vi "read_csv_StoreTrajectory_FGV.vi"(8 "Sample Time\nSeconds":dbl, 9 "inTRAJECTORY":T6 {"States"."POSE"."ROTATION"."SIN" format="%13.4f"; "States"."POSE"."ROTATION"."COS" format="%13.4f"; "States"."POSE"."ROTATION"."VALUE" format="%13.4f"; "States"."POSE"."TRANSLATION"."Y" format="%14.3f"; "States"."POSE"."TRANSLATION"."X" format="%14.3f"; "TotalTImeSecs" format="%20.3f"}, 11 "Command":T5(ring)) -> (1 "outTRAJECTORY":T6 {"States"."POSE"."ROTATION"."SIN" format="%13.4f"; "States"."POSE"."ROTATION"."COS" format="%13.4f"; "States"."POSE"."ROTATION"."VALUE" format="%13.4f"; "States"."POSE"."TRANSLATION"."Y" format="%14.3f"; "States"."POSE"."TRANSLATION"."X" format="%14.3f"; "TotalTImeSecs" format="%20.3f"}, 3 "outTrajectoryState":T1={"TimeSeconds"=0.0, "Velocity"=0.0, "Acceleration"=0.0, "POSE"={"TRANSLATION"={"X"=0.0, "Y"=0.0}, "ROTATION"={"VALUE"=0.0, "COS"=1.0, "SIN"=0.0}}, "Curvature"=0.0} {"POSE"."ROTATION"."SIN" format="%13.4f"; "POSE"."ROTATION"."COS" format="%13.4f"; "POSE"."ROTATION"."VALUE" format="%13.4f"; "POSE"."TRANSLATION"."Y" format="%14.3f"; "POSE"."TRANSLATION"."X" format="%14.3f"})   [LabVIEW 2019]
uses:
  <vilib>/Rock Robotics/WPI/ThirdParty/JAS_Junk/TrajLib/TypeDef/TRAJECTORY.ctl
  <vilib>/Rock Robotics/WPI/ThirdParty/JAS_Junk/TrajLib/TypeDef/TRAJ_STATE.ctl
  <vilib>/Rock Robotics/WPI/ThirdParty/JAS_Junk/TrajLib/TypeDef/POSE2D.ctl
  <vilib>/Rock Robotics/WPI/ThirdParty/JAS_Junk/TrajLib/TypeDef/TRANSLATION2D.ctl
  <vilib>/Rock Robotics/WPI/ThirdParty/JAS_Junk/TrajLib/TypeDef/ROTATION2D.ctl
  <vilib>/Rock Robotics/WPI/ThirdParty/JAS_Junk/TrajLib/Trajectory_Library.lvlib
panel:
  # "This is purposefully \n\nNOT re-entrant."
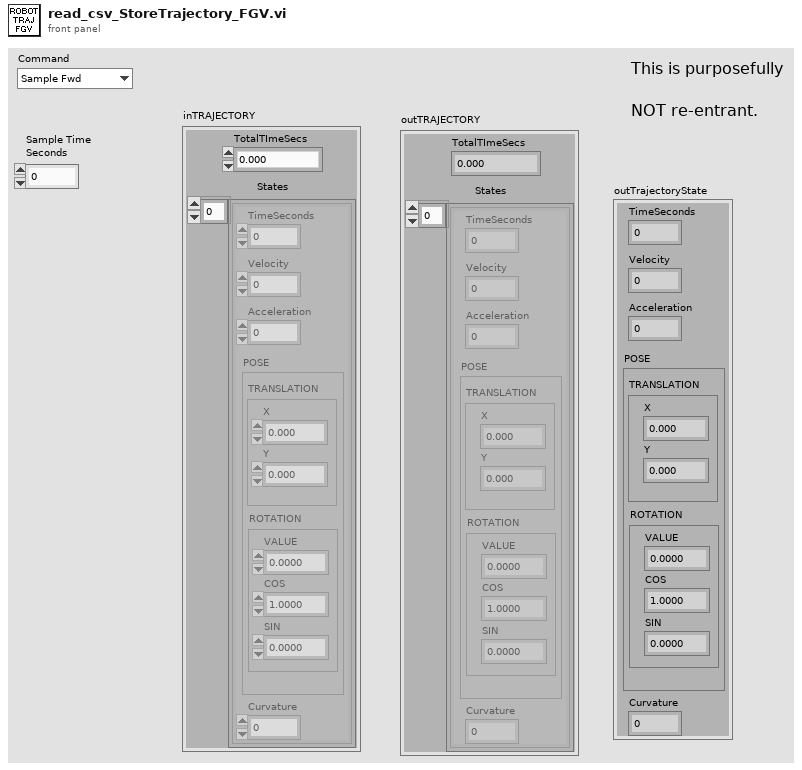
[diagram p1: front panel]
types:
  T1 = typedef "Trajectory_Library.lvlib/TRAJ_STATE.ctl" = cluster{"TimeSeconds":dbl, "Velocity":dbl, "Acceleration":dbl, "POSE":T2, "Curvature":dbl}
  T2 = typedef "Trajectory_Library.lvlib/POSE2D.ctl" = cluster{"TRANSLATION":T3, "ROTATION":T4}
  T3 = typedef "Trajectory_Library.lvlib/TRANSLATION2D.ctl" = cluster{"X":dbl, "Y":dbl}
  T4 = typedef "Trajectory_Library.lvlib/ROTATION2D.ctl" = cluster{"VALUE":dbl, "COS":dbl, "SIN":dbl}
  T5 = enum16{"Sample Fwd", "Sample Rev", "Read Traj", "Write Traj"}
  T6 = typedef "Trajectory_Library.lvlib/TRAJECTORY.ctl" = cluster{"TotalTImeSecs":dbl, "States":T1[]}
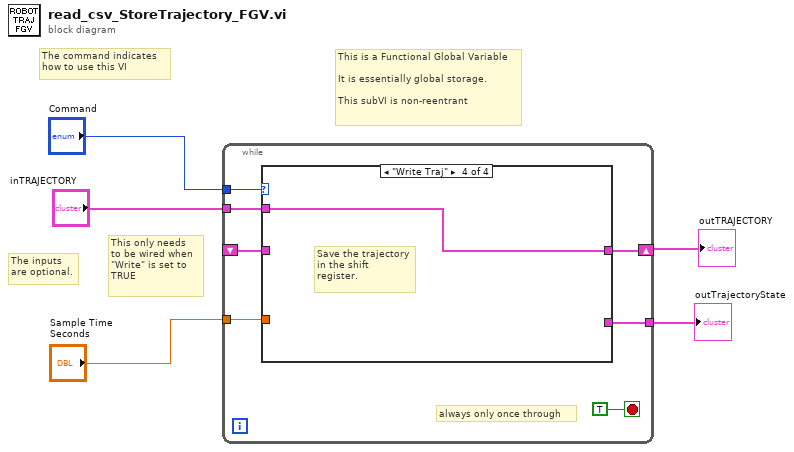
[diagram p0: block diagram]
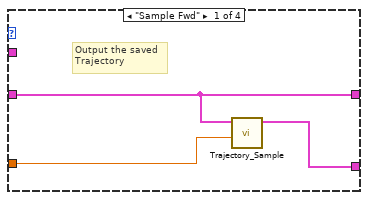
[diagram p2: hidden frame]
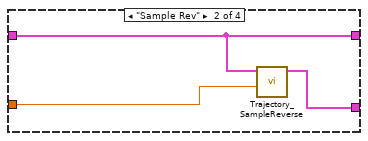
[diagram p3: hidden frame]
diagram:
  # "This only needs\nto be wired when\n\"Write\" is set to\nTRUE"
  # "The command indicates\nhow to use this VI"
  # "The inputs \nare optional."
  # "This is a Functional Global Variable\n\nIt is essentially global storage.\n\nThis subVI is non-reentrant"
  n1 = while {
    tunnel: "Command" -> [w11]
    tunnel: "inTRAJECTORY" -> [w9]
    shift-right: [w10] -> w5
    shift-left: _ -> [w8]
    tunnel: "Sample Time\nSeconds" -> [w7]
    tunnel: [w6] -> w1
    stop <- TRUE stop-if-true
    # "always only once through"
    n2 = case shown="\"Write Traj\"" w11 {
      tunnel: [w15 w18 w19 w20] -> w10
      tunnel: w9 -> [_ _ _ w20]
      tunnel: w8 -> [w15 w18 w19 _]
      tunnel: w7 -> [w14 w17 _ _]
      tunnel: [w13 w16 _ _] -> w6
      frame "Sample Fwd" {
        # "Output the saved\nTrajectory"
        n3 = call <vilib>:"Trajectory_Sample.vi"("Time"=w14, "InputTRAJECTORY"=w15) -> ("OutputTRAJ_STATE"=w13:T1)  [unwired: 9 in]
      }
      frame "Sample Rev" {
        n4 = call <vilib>:"Trajectory_SampleReverse.vi"("Time"=w17, "InputTRAJECTORY"=w18) -> ("OutputTRAJ_STATE"=w16:T1)  [unwired: 9 in]
      }
      frame "Read Traj" {
      }
      frame "Write Traj" {
        # "Save the trajectory\nin the shift \nregister."
      }
    }
  }
  "outTRAJECTORY" <- w5
  "outTrajectoryState" <- w1
